vi "TDT-Get Events Final (Tosca).vi"(0 "Data":T1={"TTankX"=refnum, "TDevAccX"=refnum, "LastTime"=0.0, "error"={"status"=FALSE, "code"=0, "source"=""}, "Block Name"="", "Circuit Tag"="", "Tank Name"="", "NumTicks"=0, "LastTick"=0.0, "Idle?"=FALSE, "Wait (ms)"=1000, "LastArtf"=0.0, "LastTosc"=0.0}, 11 "error in (no error)":errorcluster, 13 "Tetrode":bool) -> (4 "Data out":T1={"TTankX"=refnum, "TDevAccX"=refnum, "LastTime"=0.0, "error"={"status"=FALSE, "code"=0, "source"=""}, "Block Name"="", "Circuit Tag"="", "Tank Name"="", "NumTicks"=0, "LastTick"=0.0, "Idle?"=FALSE, "Wait (ms)"=1000, "LastArtf"=0.0, "LastTosc"=0.0}, 8 "Events":dbl[][](array[numeric]), 10 "total ticks":i32, 15 "error out":errorcluster)   [LabVIEW 2015]
uses:
  TDT Interface Data.ctl
panel:
  out "NumTicks":i32
  in  "Poll Interval (s)":dbl=2.0
  in  "Timeout (s)":dbl=10.0
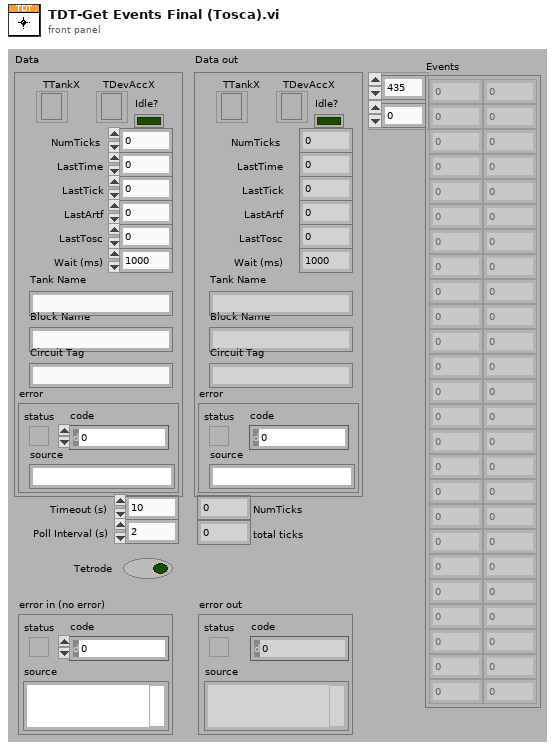
[diagram p1: front panel]
types:
  T1 = typedef "TDT Interface Data.ctl" = cluster{"TTankX":refnum<k7>, "TDevAccX":refnum<k7>, "LastTime":dbl, "error":errorcluster, "Block Name":string, "Circuit Tag":string, "Tank Name":string, "NumTicks":i32, "LastTick":dbl, "Idle?":bool, "Wait (ms)":u32, "LastArtf":dbl, "LastTosc":dbl}
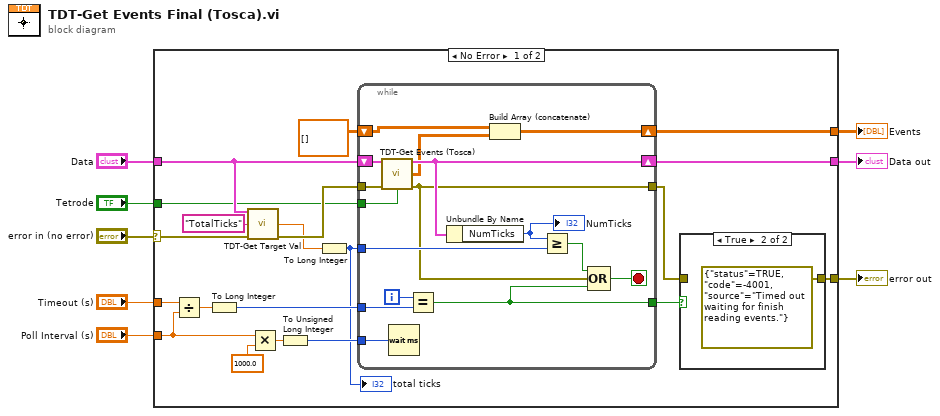
[diagram p0: block diagram]
diagram:
  n1 = case shown="No Error" "error in (no error)" {
    selector: "error in (no error)" -> [w14 w48]
    tunnel: [w20 w48] -> w7
    tunnel: "Data" -> [w11 w47]
    tunnel: "Timeout (s)" -> [w25 _]
    tunnel: "Poll Interval (s)" -> [w24 _]
    tunnel: [w17 w47] -> w3
    tunnel: [w16 _] -> w2
    tunnel: "Tetrode" -> [w9 _]
    frame No Error {
      n2 = Divide(x=w25, y=w24) -> (x/y=w28:dbl)
      n3 = To Long Integer(number=w28) -> (32bit integer=w22:i32)
      n4 = call "TDT-Get Target Val.vi"("Data"=w11, "Target"="TotalTicks", "error in (no error)"=w14) -> ("GetTargetVal"=w12:dbl, "error out"=w13:errorcluster)  [unwired: 11 in]
      n5 = Multiply(x=w24, y=1000.0) -> (x*y=w27:dbl)
      n6 = To Unsigned Long Integer(number=w27) -> (unsigned 32bit integer=w23:u32)
      n7 = To Long Integer(number=w12) -> (32bit integer=w19:i32)
      "total ticks" <- w19
      n8 = while {
        tunnel: w13 -> [w39]
        tunnel: w23 -> [w45]
        tunnel: w22 -> [w43]
        tunnel: [w41] -> w21
        tunnel: w19 -> [w36]
        shift-right: [w38] -> w17
        shift-left: w11 -> [w40]
        tunnel: [w32] -> w18
        shift-right: [w34] -> w16
        shift-left: dbl[][] [] -> [w33]
        tunnel: w9 -> [w31]
        i -> [w44]
        stop <- w46 stop-if-true
        n9 = call "TDT-Get Events (Tosca).vi"("Data"=w40, "error in (no error)"=w39, "Tetrode"=w31) -> ("Data out"=w38:T1, "Events"=w35:dbl[][], "error out"=w32:errorcluster)  [unwired: 10 in]
        n10 = Wait (ms)(milliseconds to wait=w45) -> ()  [unwired: 1 out]
        n11 = Equal?(x=w44, y=w43) -> (x = y?=w41:bool)
        n12 = Unbundle By Name(w38) -> ("NumTicks"=w37:i32)
        "NumTicks" <- w37
        n13 = Build Array (concatenate)(w33, w35) -> (w34:dbl[][])
        n14 = Greater Or Equal?(x=w37, y=w36) -> (x >= y?=w42:bool)
        n15 = Compound Arithmetic op=OR(w42, w32, w41) -> (w46:bool)
      }
      n16 = case shown="True" w21 {
        tunnel: [w29 errorcluster {"status"=TRUE, "code"=-4001, "source"="Timed out waiting for finish reading events."} ("error out")] -> w20
        tunnel: w18 -> [w29 _]
        frame False {
        }
        frame True {
        }
      }
    }
    frame Error {
    }
  }
  "error out" <- w7
  "Data out" <- w3
  "Events" <- w2
